vi "Práctica 1.vi"() -> ()   [LabVIEW 2015]
panel:
  out "Q4":bool
  out "Q3":bool
  out "Q2":bool
  out "Q1":bool
  in  "I5":bool
  in  "I4":bool
  in  "I3":bool
  in  "I2":bool
  in  "I1":bool
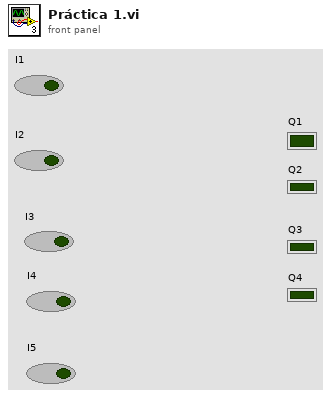
[diagram p1: front panel]
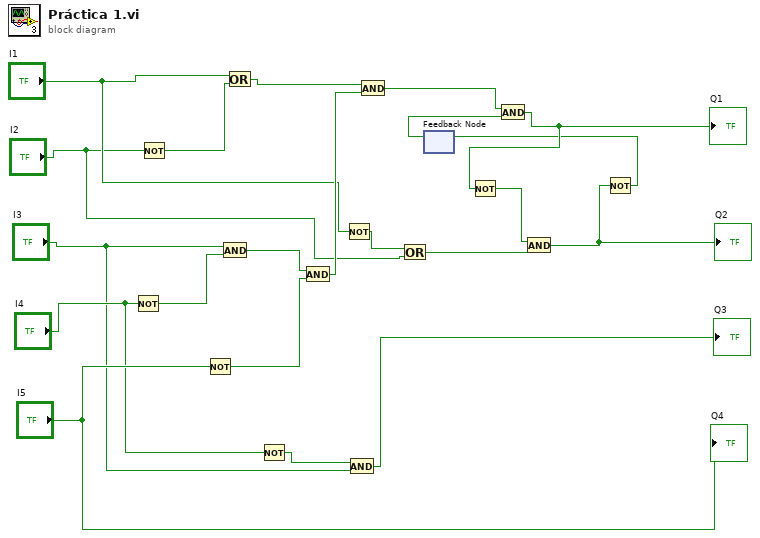
[diagram p0: block diagram]
diagram:
  n1 = Not(x="I4") -> (.not. x?=w18:bool)
  n2 = Not(x="I2") -> (.not. x?=w21:bool)
  n3 = Not(x="I5") -> (.not. x?=w16:bool)
  n4 = And(x="I3", y=w18) -> (x .and. y?=w17:bool)
  n5 = Or(x="I1", y=w21) -> (x .or. y?=w20:bool)
  n6 = Not(x="I4") -> (.not. x?=w4:bool)
  n7 = And(x=w17, y=w16) -> (x .and. y?=w14:bool)
  n8 = Not(x="I1") -> (.not. x?=w13:bool)
  n9 = And(x=w4, y="I3") -> (x .and. y?=→"Q3":bool)
  n10 = And(x=w20, y=w14) -> (x .and. y?=w19:bool)
  n11 = Or(x=w13, y="I2") -> (x .or. y?=w10:bool)
  n12 = feedback #1() -> (w5:bool)  [unwired: 1 in]
  n13 = And(x=w19, y=w5) -> (x .and. y?=w9:bool)
  "Q1" <- w9
  n14 = Not(x=w9) -> (.not. x?=w8:bool)
  n15 = And(x=w8, y=w10) -> (x .and. y?=w7:bool)
  "Q2" <- w7
  n16 = Not(x=w7) -> (.not. x?=w6:bool)
  n17 = feedback-in #1(w6) -> ()
  "Q4" <- "I5"
